vi "PhotonCamera_GetPipelineIndex.vi"(11 "CameraName":string) -> (3 "PipelineIndex":i32)   [LabVIEW 2019, in "PhotonVisionLib.lvlib"]
doc: "Returns the active pipeline index.\n\nInputs:\n - cameraName -- The nickname of the camera (found in the PhotonVision UI).\n \nOutputs:\n - PipelineIndex -- Active Pipeline Index"
uses:
  PhotonVisionLib.lvlib
  <vilib>/Rock Robotics/Network Tables/NT Read Number.vi
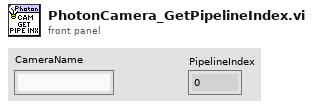
[diagram p1: front panel]
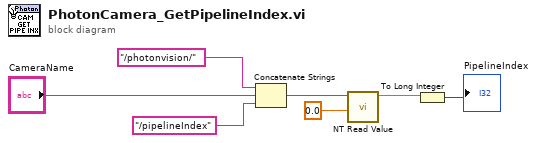
[diagram p0: block diagram]
diagram:
  n1 = Concatenate Strings("/photonvision/", "CameraName", "/pipelineIndex") -> (w4:string)
  n2 = call-poly <vilib>:"NT Read Value.vi"("Default Value"=0.0, "Name"=w4) -> ("Numeric"=w1:dbl)  [unwired: 8 in, 1 out]
  n3 = To Long Integer(number=w1) -> (32bit integer=→"PipelineIndex":i32)
